vi "Synchronized DELETE Generic.vi"(0 "DEL VI Reference":refnum<vi>) -> ()   [LabVIEW 2013]
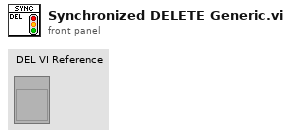
[diagram p1: front panel]
types:
  T1 = typedef "Semaphore RefNum" = refnum<k1>
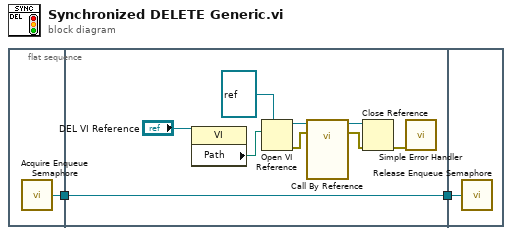
[diagram p0: block diagram]
diagram:
  n1 = flat-sequence {
    tunnel: [w3] -> w2
    tunnel: w2 -> [w12]
    tunnel: [w12] -> w1
    tunnel: w1 -> [w13]
    frame #0 {
      n2 = call "Acquire Enqueue Semaphore.vi"() -> ("Semaphore Reference"=w3:T1)
    }
    frame #1 {
      n3 = property class="VI"(reference="DEL VI Reference") -> ("Path"=w9:path)  [unwired: 1 in, 2 out]
      n4 = Open VI Reference(type specifier VI Refnum (for type only)=refnum<vi> refnum, vi path=w9) -> (vi reference=w8:refnum<vi>, error out=w7:errorcluster)  [unwired: 4 in]
      n5 = call-by-ref "?"(reference=w8, error in=w7) -> (reference out=w6:refnum<vi>, error out=w5:errorcluster)  [unwired: 1 in]
      n6 = Close Reference(reference=w6, error in (no error)=w5) -> (error out=w4:errorcluster)
      n7 = call <vilib>:"Simple Error Handler.vi"("error in (no error)"=w4) -> ()  [unwired: 4 in, 5 out]
    }
    frame #2 {
      n8 = call "Release Enqueue Semaphore.vi"("Semaphore Reference"=w13) -> ()
    }
  }
